vi "Configure Width Trigger Source [WT] Core.vi"(0 "CS++Scope":refnum<class "CS++Scope.lvclass">, 1 "trigger source (\"CHANNEL1\")":string(combo)="CHANNEL1", 2 "trigger level (0.0 V)":dbl[unit] format="%.3f", 3 "width condition (Within)":i32(ring)=1 items=["Within"=1, "Outside"=2], 4 "width polarity (Positive)":i32(ring)=1 items=["Positive"=1, "Negative"=2], 5 "error in (no error)":errorcluster, 6 "width low threshold (1.0 E-9 V)":dbl[unit]=1e-09 format="%^.3e", 8 "width high threshold (2.0 E-9 V)":dbl[unit]=2e-09 format="%^.3e") -> (14 "CS++Scope out":refnum<class "CS++Scope.lvclass">, 19 "error out":errorcluster)   [LabVIEW 2013, in "CS++Scope.lvlib" / "CS++Scope.lvclass"]
doc: "This VI configures the width trigger. A width trigger occurs when the oscilloscope detects a positive or negative pulse with a width between, or optionally outside, the width thresholds. You specify the width thresholds with the Width Low Threshold and Width High Threshold parameters. You specify whether the oscilloscope triggers on pulse widths that are within or outside the width thresholds with the Width Condition parameter. You specify the polarity of the pulse with the Width Polarity parameter. The trigger does not actually occur until the edge of a pulse that corresponds to the Width Low Threshold, Width High Threshold, Width Condition, and Width Polarity crosses the threshold you specify in the Trigger Level parameter.\n\nNote (1) This VI affects instrument behavior only if the trigger type is IVISCOPE_VAL_WIDTH_TRIGGER. Call the IviScope Configure Trigger and IviScope Configure Trigger Coupling VIs to set the trigger type and trigger coupling before calling this VI.\n(2) This VI is part of the IviScopeWidthTrigger [WT] extension group."
uses:
  CS++Scope.lvclass
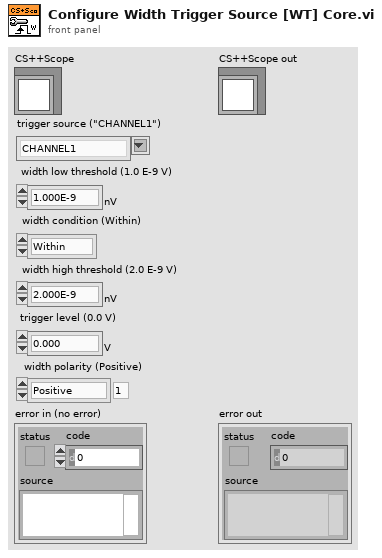
[diagram p1: front panel]
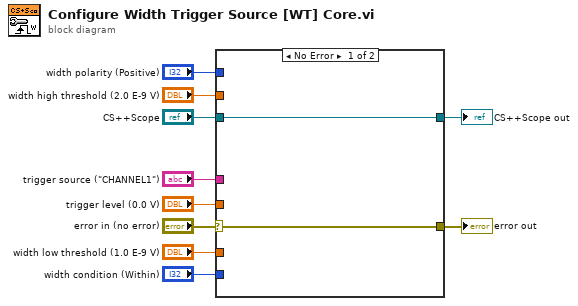
[diagram p0: block diagram]
diagram:
  n1 = case shown="No Error" "error in (no error)" {
    selector: "error in (no error)" -> [w12 w14]
    tunnel: [w12 w14] -> w9
    tunnel: [w11 w13] -> w1
    tunnel: "CS++Scope" -> [w11 w13]
    tunnel: "trigger source (\"CHANNEL1\")" -> [_ _]
    tunnel: "trigger level (0.0 V)" -> [_ _]
    tunnel: "width low threshold (1.0 E-9 V)" -> [_ _]
    tunnel: "width condition (Within)" -> [_ _]
    tunnel: "width high threshold (2.0 E-9 V)" -> [_ _]
    tunnel: "width polarity (Positive)" -> [_ _]
    frame No Error {
    }
    frame Error {
    }
  }
  "error out" <- w9
  "CS++Scope out" <- w1
